vi "acquireValue.vi"(8 "error in (no error)":errorcluster, 10 "nextSample?":bool, 11 "startScanDt in":refnum<class "startScanDt.lvclass">) -> (0 "error out":errorcluster, 1 "function return":i32, 2 "variantData":variant, 3 "startScanDt out":refnum<class "startScanDt.lvclass">)   [LabVIEW 2016, in "SALLV_MtAtElectrometer_Messaging.lvlib" / "startScanDt.lvclass"]
uses:
  startScanDt.lvclass
  ts_sallv_MtAtElectrometer/SALLV_MtAtElectrometer.lvlib
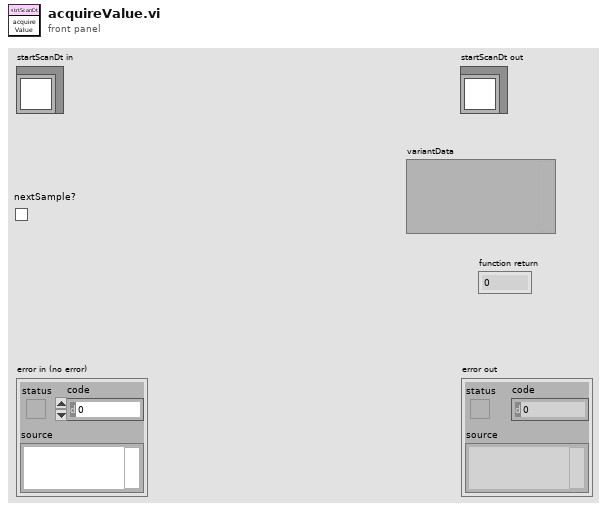
[diagram p1: front panel]
types:
  T1 = typedef "SALLV_MtAtElectrometer.lvlib/command_startScanDt.ctl" = cluster{"scanDuration":sgl}
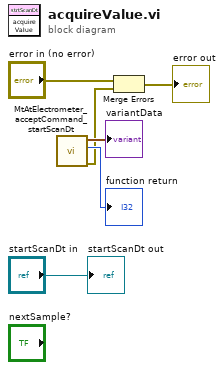
[diagram p0: block diagram]
diagram:
  n1 = call "MtAtElectrometer_acceptCommand_startScanDt.vi"() -> ("error out"=w1:errorcluster, "function return"=→"function return":i32, "command_startScanDt_Ctl out"=→"variantData":T1)  [unwired: 9 in]
  n2 = Merge Errors("error in (no error)", w1) -> (→"error out":errorcluster)
  "startScanDt out" <- "startScanDt in"
